vi "Camera1.vi"() -> ()   [LabVIEW 2020]
uses:
  Control 1.ctl
panel:
  in  "Frame for delta T":i32
  out "Delta T image":dbl[][](graph)
  out "Delta T":dbl[][][](array[numeric])
  out "FrameData even":dbl[][][](array[numeric])
  out "FrameData odd":dbl[][][](array[numeric])
  out "FrameData":dbl[][][](array[numeric])
  out "ExtChData":dbl[][](array[numeric])
  in  "Timeout":i32
  in  "ExChs":i32
  in  "Frames":T1=1
  in  "Acq Trigger?":bool
  in  "Offset":i32=128 min=0 max=255 step=1
  out "Actual (us)":dbl
  in  "IntegrationTime (us)":dbl=1.0 min=0.1 max=5000.0 step=0.1
  out "MaxFrameRate":dbl
  in  "Frame Size (Row x Col)":u16(ring) items=["128x128", "96x128", "64x128", "32x128"]
  out "TempK":dbl
  out "First Image":dbl[][](graph)
  out "error":errorcluster
  # "IMAGE SETTINGS"
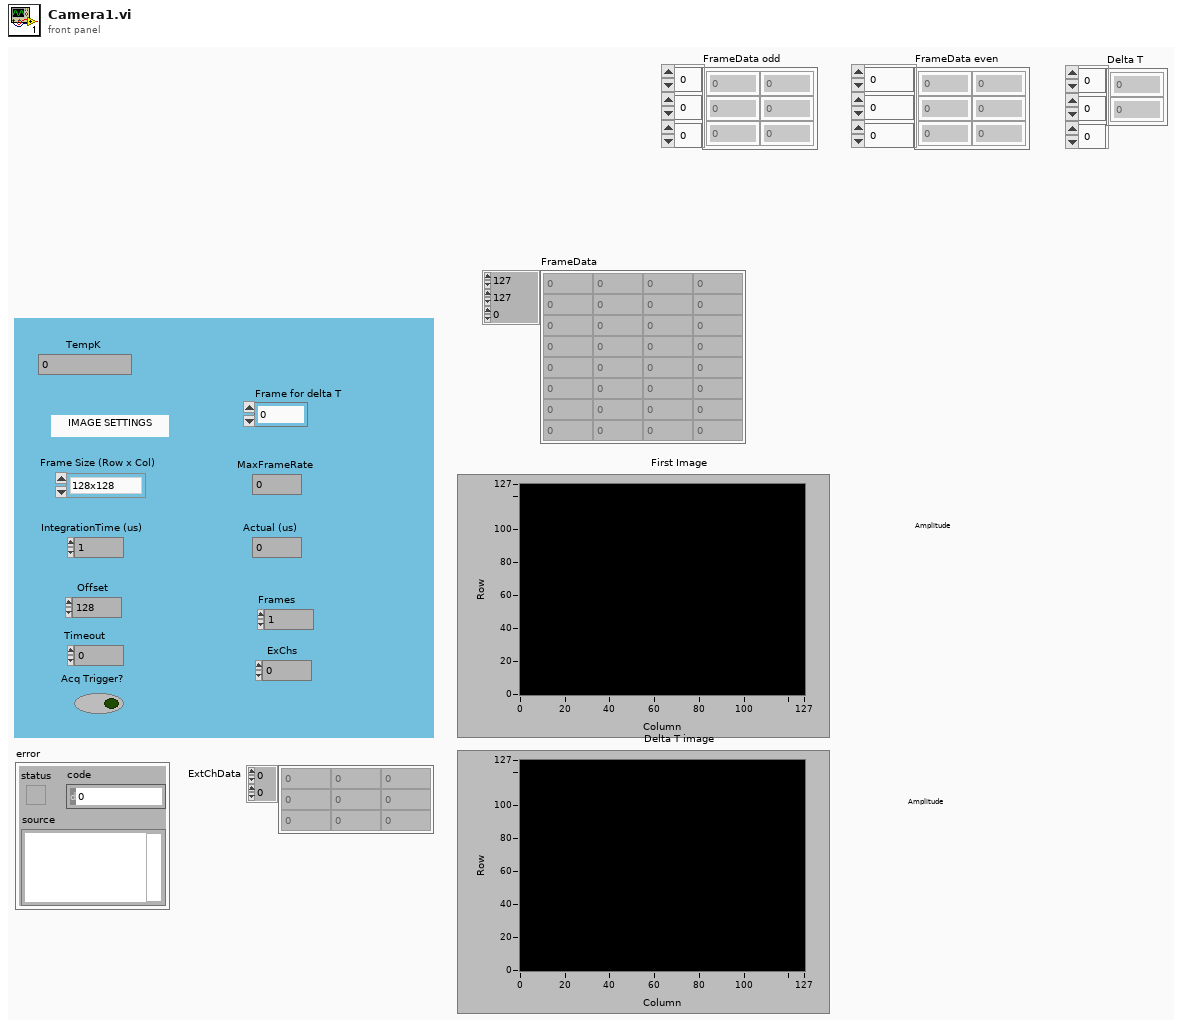
[diagram p1: front panel]
types:
  T1 = typedef "Control 1.ctl" = i32
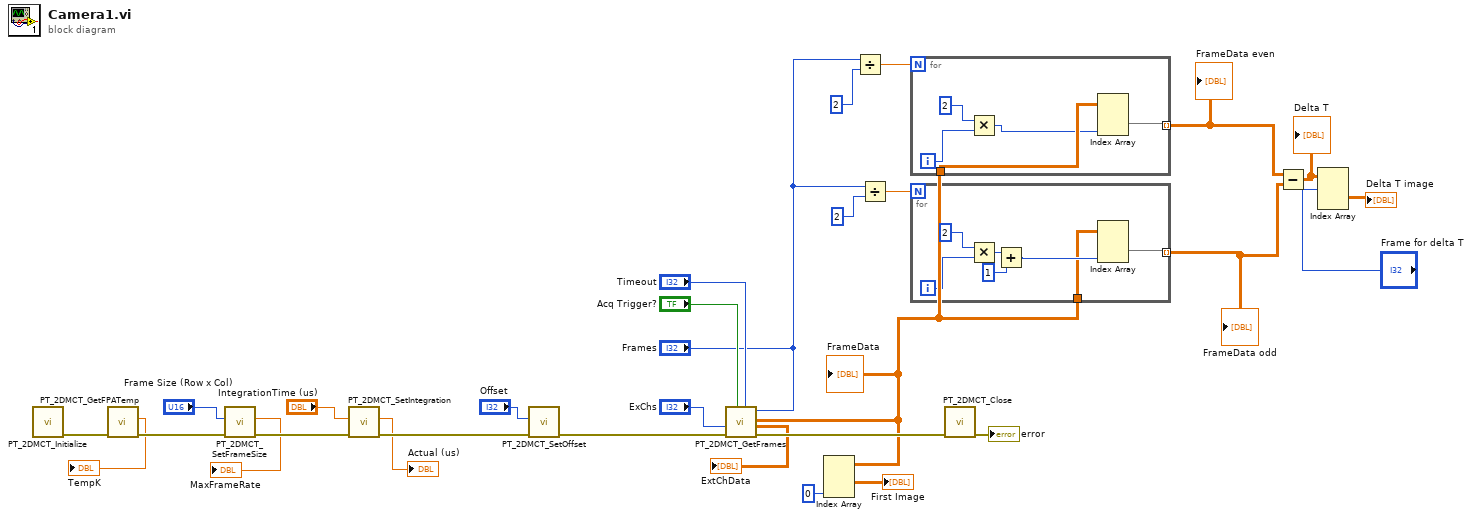
[diagram p0: block diagram]
diagram:
  n1 = call "PT_2DMCT_Initialize.vi"() -> ("error out"=w26:errorcluster)  [unwired: 11 in]
  n2 = call "PT_2DMCT_GetFPATemp.vi"("error in (no error)"=w26) -> ("error out"=w25:errorcluster, "TempK"=→"TempK":dbl)  [unwired: 8 in, 1 out]
  n3 = call "PT_2DMCT_SetFrameSize.vi"("error in (no error)"=w25, "Frame Size (Row x Col)"="Frame Size (Row x Col)") -> ("error out"=w24:errorcluster, "MaxFrameRate"=→"MaxFrameRate":dbl)  [unwired: 4 in]
  n4 = call "PT_2DMCT_SetIntegration.vi"("error in (no error)"=w24, "IntegrationTime (us)"="IntegrationTime (us)") -> ("error out"=w23:errorcluster, "Actual (us)"=→"Actual (us)":dbl)  [unwired: 4 in]
  n5 = call "PT_2DMCT_SetOffset.vi"("error in (no error)"=w23, "Offset"="Offset") -> ("error out"=w22:errorcluster)  [unwired: 9 in]
  n6 = call "PT_2DMCT_GetFrames.vi"("Timeout"="Timeout", "Acq Trigger?"="Acq Trigger?", "error in (no error)"=w22, "ExChs"="ExChs", "Frames"="Frames") -> ("error out"=w28:errorcluster, "ExtChData"=→"ExtChData":dbl[][], "FrameData"=w6:dbl[][][])  [unwired: 4 in]
  "FrameData" <- w6
  n7 = Index Array(array=w6, index (dim 2)=0 ("disabled index (col)")) -> (element=→"First Image":dbl[][])  [unwired: 2 in]
  n8 = Divide(x="Frames", y=T1 2) -> (x/y=w8:dbl)
  n9 = Divide(x="Frames", y=T1 2) -> (x/y=w10:dbl)
  n10 = for {
    N: w8 -> [_]
    tunnel: [w33] -> w3 mode=indexing
    tunnel: w6 -> [w32]
    i -> [w35]
    n11 = Multiply(x=2, y=w35) -> (x*y=w31:i32)
    n12 = Index Array(array=w32, index (dim 2)=w31) -> (element=w33:dbl[][])  [unwired: 2 in]
  }
  "FrameData even" <- w3
  n13 = for {
    N: w10 -> [_]
    tunnel: w6 -> [w37]
    tunnel: [w36] -> w2 mode=indexing
    i -> [w42]
    n14 = Multiply(x=2, y=w42) -> (x*y=w40:i32)
    n15 = Add(x=w40, y=1) -> (x+y=w38:i32)
    n16 = Index Array(array=w37, index (dim 2)=w38) -> (element=w36:dbl[][])  [unwired: 2 in]
  }
  "FrameData odd" <- w2
  n17 = call "PT_2DMCT_Close.vi"("error in (no error)"=w28) -> ("error out"=→"error":errorcluster)  [unwired: 10 in]
  n18 = Subtract(x=w3, y=w2) -> (x-y=w5:dbl[][][])
  "Delta T" <- w5
  n19 = Index Array(array=w5, index (dim 0)="Frame for delta T") -> (element=→"Delta T image":dbl[][])  [unwired: 2 in]
